vi "AcquireImage.vi"(8 "error in":errorcluster, 11 "Session In":T2) -> (0 "error out":errorcluster, 2 "Image":T1(plugin-control), 3 "Session Out":T2)   [LabVIEW 2017]
uses:
  <vilib>/userdefined/High Color/IMAQdx.ctl
  <vilib>/vision/driver/NI_Vision_Acquisition_Software.lvlib
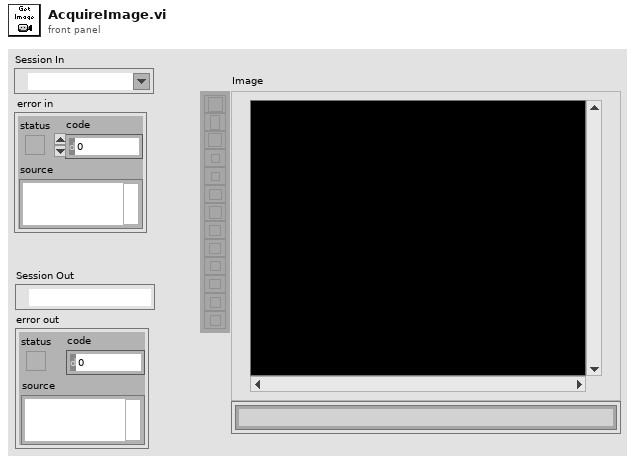
[diagram p1: front panel]
types:
  T1 = typedef "IMAQ Image.ctl" = refnum<image>
  T2 = typedef "IMAQdx.ctl" = refnum<k21>
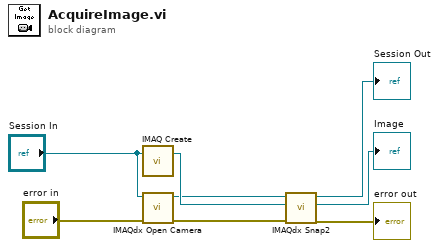
[diagram p0: block diagram]
diagram:
  n1 = call "IMAQ Create"("Image Name"="Session In") -> ("New Image"=w7:T1)  [unwired: 4 in, 1 out]
  n2 = call <vilib>:"IMAQdx Open Camera.vi"("error in"="error in", "Session In"="Session In") -> ("error out"=w3:errorcluster, "Session Out"=w6:T2)  [unwired: 8 in]
  n3 = call <vilib>:"IMAQdx Snap2.vi"("error in"=w3, "Image In"=w7, "Session In"=w6) -> ("error out"=→"error out":errorcluster, "Image Out"=→"Image":T1, "Session Out"=→"Session Out":T2)  [unwired: 6 in]
